vi "FilterBySize.vi"(10 "Size":T1, 11 "Products In":refnum<class "Product.lvclass">[](array[class])) -> (3 "Filtered Products":refnum<class "Product.lvclass">[](array[class]))   [LabVIEW 2018, in "ProductFilter.lvclass"]
uses:
  ProductFilter.lvclass
  Product/Product.lvclass
  Product/Size.ctl
  Product/Product.lvclass/Product.ctl
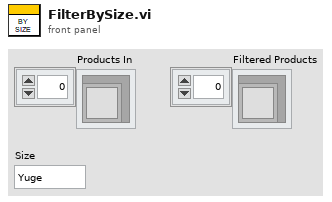
[diagram p1: front panel]
types:
  T1 = typedef "Product.lvclass/Size.ctl" = enum16{"Yuge", "Big", "Medium", "Small"}
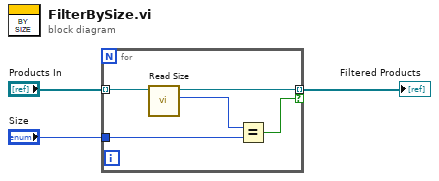
[diagram p0: block diagram]
diagram:
  n1 = for {
    tunnel: "Products In" -> [w6] mode=indexing
    tunnel: [w5] -> w2 mode=indexing if=w7
    tunnel: "Size" -> [w8]
    n2 = call "Read Size.vi"("Product In"=w6) -> ("Size"=w4:T1, "Product Out"=w5:refnum<class "Product.lvclass">)  [unwired: 9 in]
    n3 = Equal?(x=w4, y=w8) -> (x = y?=w7:bool)
  }
  "Filtered Products" <- w2
